vi "NMD Analysis 3.1.vi"(8 "error in (no error)":errorcluster, 11 "Data Cluster In":T1={"Selected File"=path "", "Full Text File"=[], "Data Array"=[], "Times Array"=[], "Sensor Array"=[], "Subset Array"=[], "Smoothness Values"=[], "Sensor Select 1"=refnum, "Sensor Select 2"=refnum, "Sensor Select 3"=refnum, "Sensor Select 4"=refnum, "Start Times"=[], "End Times"=[], "Cursor List"=[{"Name"="Event Marker          ", "Color"=16777200, "Style"=0, "Point Style"=0, "Name Visible"=FALSE, "Allow Drag"=FALSE, "Cursor Mode"=0, "Plot"=0, "Index"=0, "Position"={"X"=4.0, "Y"=1.0}, "X Scale"=0, "Y Scale"=0, "Watch Plots"=[], "Watch All Plots"=FALSE, "Plot Area"=0, "Label Offset"={"X"=-50.0, "Y"=150.0}}, {"Name"="Upper Sensor", "Color"=13816500, "Style"=6, "Point Style"=0, "Name Visible"=FALSE, "Allow Drag"=FALSE, "Cursor Mode"=0, "Plot"=0, "Index"=0, "Position"={"X"=-1.0, "Y"=5.0}, "X Scale"=0, "Y Scale"=0, "Watch Plots"=[], "Watch All Plots"=FALSE, "Plot Area"=0, "Label Offset"={"X"=0.0, "Y"=0.0}}, {"Name"="Lower Sensor", "Color"=13816500, "Style"=6, "Point Style"=0, "Name Visible"=FALSE, "Allow Drag"=FALSE, "Cursor Mode"=0, "Plot"=0, "Index"=0, "Position"={"X"=-1.0, "Y"=30.0}, "X Scale"=0, "Y Scale"=0, "Watch Plots"=[], "Watch All Plots"=FALSE, "Plot Area"=0, "Label Offset"={"X"=0.0, "Y"=0.0}}], "Listbox 1"=refnum, "Listbox 2"=refnum, "Listbox 3"=refnum, "Listbox 4"=refnum, "Labels"=["Why", "is", "this", "still", "not", "built", "into", "Labview?", "This", "is", "shameful."], "Event Array"=[], "Event Names"=[], "Event Times"=[], "Save Plot Button"=refnum, "Sensor Plot Refs"=[], "Selected Event (Title)"="", "Upper Cursor"=0.0, "Lower Cursor"=0.0, "Z Max"=0.0, "Z Min"=0.0}) -> (0 "error out":errorcluster, 3 "Data Cluster Out":T1={"Selected File"=path "", "Full Text File"=[], "Data Array"=[], "Times Array"=[], "Sensor Array"=[], "Subset Array"=[], "Smoothness Values"=[], "Sensor Select 1"=refnum, "Sensor Select 2"=refnum, "Sensor Select 3"=refnum, "Sensor Select 4"=refnum, "Start Times"=[], "End Times"=[], "Cursor List"=[{"Name"="Event Marker          ", "Color"=16777200, "Style"=0, "Point Style"=0, "Name Visible"=FALSE, "Allow Drag"=FALSE, "Cursor Mode"=0, "Plot"=0, "Index"=0, "Position"={"X"=4.0, "Y"=1.0}, "X Scale"=0, "Y Scale"=0, "Watch Plots"=[], "Watch All Plots"=FALSE, "Plot Area"=0, "Label Offset"={"X"=-50.0, "Y"=150.0}}, {"Name"="Upper Sensor", "Color"=13816500, "Style"=6, "Point Style"=0, "Name Visible"=FALSE, "Allow Drag"=FALSE, "Cursor Mode"=0, "Plot"=0, "Index"=0, "Position"={"X"=-1.0, "Y"=5.0}, "X Scale"=0, "Y Scale"=0, "Watch Plots"=[], "Watch All Plots"=FALSE, "Plot Area"=0, "Label Offset"={"X"=0.0, "Y"=0.0}}, {"Name"="Lower Sensor", "Color"=13816500, "Style"=6, "Point Style"=0, "Name Visible"=FALSE, "Allow Drag"=FALSE, "Cursor Mode"=0, "Plot"=0, "Index"=0, "Position"={"X"=-1.0, "Y"=30.0}, "X Scale"=0, "Y Scale"=0, "Watch Plots"=[], "Watch All Plots"=FALSE, "Plot Area"=0, "Label Offset"={"X"=0.0, "Y"=0.0}}], "Listbox 1"=refnum, "Listbox 2"=refnum, "Listbox 3"=refnum, "Listbox 4"=refnum, "Labels"=["Why", "is", "this", "still", "not", "built", "into", "Labview?", "This", "is", "shameful."], "Event Array"=[], "Event Names"=[], "Event Times"=[], "Save Plot Button"=refnum, "Sensor Plot Refs"=[], "Selected Event (Title)"="", "Upper Cursor"=0.0, "Lower Cursor"=0.0, "Z Max"=0.0, "Z Min"=0.0})   [LabVIEW 2020]
uses:
  Controls/DataCluster.ctl
  <vilib>/Utility/miscctls.llb/LVCursorListTypeDef.ctl
  Controls/SPARC Analysis States.ctl
  <userlib>/_OpenG.lib/file/file.llb/File Exists - Scalar__ogtk.vi
panel:
  out "NMD Plot":picture
  out "Saving":bool
  out "Analyzing":bool
  out "Segmenting":bool
  out "Selected Segment":dbl[][](graph)
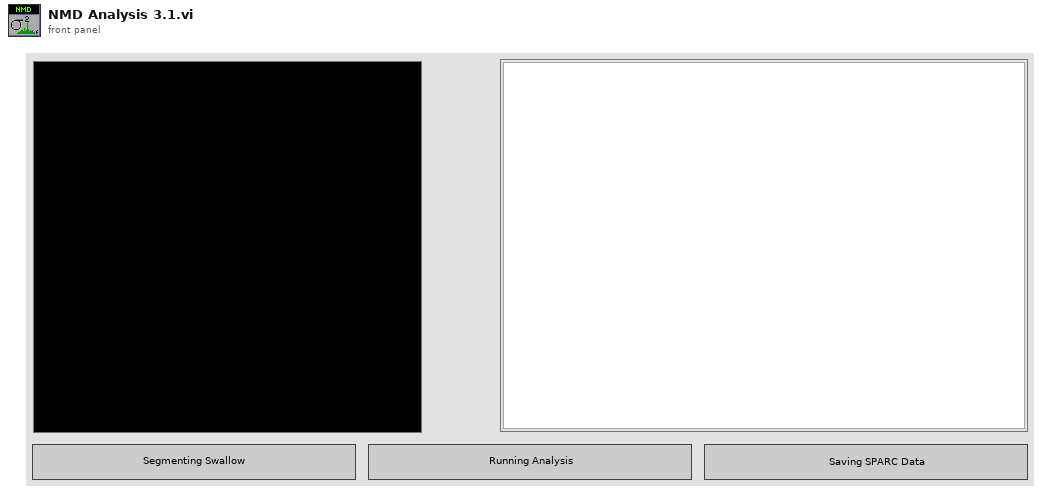
[diagram p1: front panel]
types:
  T1 = typedef "DataCluster.ctl" = cluster{"Selected File":path, "Full Text File":string[][], "Data Array":dbl[][], "Times Array":dbl[], "Sensor Array":dbl[], "Subset Array":dbl[][], "Smoothness Values":dbl[], "Sensor Select 1":refnum<vi>, "Sensor Select 2":refnum<vi>, "Sensor Select 3":refnum<vi>, "Sensor Select 4":refnum<vi>, "Start Times":dbl[], "End Times":dbl[], "Cursor List":T2, "Listbox 1":refnum<vi>, "Listbox 2":refnum<vi>, "Listbox 3":refnum<vi>, "Listbox 4":refnum<vi>, "Labels":string[], "Event Array":dbl[][], "Event Names":string[], "Event Times":dbl[], "Save Plot Button":refnum<vi>, "Sensor Plot Refs":refnum<vi>[], "Selected Event (Title)":string, "Upper Cursor":dbl, "Lower Cursor":dbl, "Z Max":dbl, "Z Min":dbl}
  T2 = typedef "LVCursorListTypeDef.ctl" = cluster{"Name":string, "Color":u32, "Style":u8, "Point Style":u8, "Name Visible":bool, "Allow Drag":bool, "Cursor Mode":u32, "Plot":i32, "Index":i32, "Position":cluster{"X":dbl, "Y":dbl}, "X Scale":u32, "Y Scale":u32, "Watch Plots":i32[], "Watch All Plots":bool, "Plot Area":i32, "Label Offset":cluster{"X":dbl, "Y":dbl}}[]
  T3 = typedef "SPARC Analysis States.ctl" = enum16{"Segment", "Analyze", "Save"}
  T4 = cluster{"Cursor List[0]":cluster{"Name":string, "Color":u32, "Style":u8, "Point Style":u8, "Name Visible":bool, "Allow Drag":bool, "Cursor Mode":u32, "Plot":i32, "Index":i32, "Position":cluster{"X":dbl, "Y":dbl}, "X Scale":u32, "Y Scale":u32, "Watch Plots":i32[], "Watch All Plots":bool, "Plot Area":i32, "Label Offset":cluster{"X":dbl, "Y":dbl}}, "Cursor List[1]":cluster{"Name":string, "Color":u32, "Style":u8, "Point Style":u8, "Name Visible":bool, "Allow Drag":bool, "Cursor Mode":u32, "Plot":i32, "Index":i32, "Position":cluster{"X":dbl, "Y":dbl}, "X Scale":u32, "Y Scale":u32, "Watch Plots":i32[], "Watch All Plots":bool, "Plot Area":i32, "Label Offset":cluster{"X":dbl, "Y":dbl}}, "Cursor List[2]":cluster{"Name":string, "Color":u32, "Style":u8, "Point Style":u8, "Name Visible":bool, "Allow Drag":bool, "Cursor Mode":u32, "Plot":i32, "Index":i32, "Position":cluster{"X":dbl, "Y":dbl}, "X Scale":u32, "Y Scale":u32, "Watch Plots":i32[], "Watch All Plots":bool, "Plot Area":i32, "Label Offset":cluster{"X":dbl, "Y":dbl}}, "Cursor List[3]":cluster{"Name":string, "Color":u32, "Style":u8, "Point Style":u8, "Name Visible":bool, "Allow Drag":bool, "Cursor Mode":u32, "Plot":i32, "Index":i32, "Position":cluster{"X":dbl, "Y":dbl}, "X Scale":u32, "Y Scale":u32, "Watch Plots":i32[], "Watch All Plots":bool, "Plot Area":i32, "Label Offset":cluster{"X":dbl, "Y":dbl}}, "Cursor List[4]":cluster{"Name":string, "Color":u32, "Style":u8, "Point Style":u8, "Name Visible":bool, "Allow Drag":bool, "Cursor Mode":u32, "Plot":i32, "Index":i32, "Position":cluster{"X":dbl, "Y":dbl}, "X Scale":u32, "Y Scale":u32, "Watch Plots":i32[], "Watch All Plots":bool, "Plot Area":i32, "Label Offset":cluster{"X":dbl, "Y":dbl}}, "Cursor List[5]":cluster{"Name":string, "Color":u32, "Style":u8, "Point Style":u8, "Name Visible":bool, "Allow Drag":bool, "Cursor Mode":u32, "Plot":i32, "Index":i32, "Position":cluster{"X":dbl, "Y":dbl}, "X Scale":u32, "Y Scale":u32, "Watch Plots":i32[], "Watch All Plots":bool, "Plot Area":i32, "Label Offset":cluster{"X":dbl, "Y":dbl}}, "Cursor List[6]":cluster{"Name":string, "Color":u32, "Style":u8, "Point Style":u8, "Name Visible":bool, "Allow Drag":bool, "Cursor Mode":u32, "Plot":i32, "Index":i32, "Position":cluster{"X":dbl, "Y":dbl}, "X Scale":u32, "Y Scale":u32, "Watch Plots":i32[], "Watch All Plots":bool, "Plot Area":i32, "Label Offset":cluster{"X":dbl, "Y":dbl}}, "Cursor List[7]":cluster{"Name":string, "Color":u32, "Style":u8, "Point Style":u8, "Name Visible":bool, "Allow Drag":bool, "Cursor Mode":u32, "Plot":i32, "Index":i32, "Position":cluster{"X":dbl, "Y":dbl}, "X Scale":u32, "Y Scale":u32, "Watch Plots":i32[], "Watch All Plots":bool, "Plot Area":i32, "Label Offset":cluster{"X":dbl, "Y":dbl}}, "Cursor List[8]":cluster{"Name":string, "Color":u32, "Style":u8, "Point Style":u8, "Name Visible":bool, "Allow Drag":bool, "Cursor Mode":u32, "Plot":i32, "Index":i32, "Position":cluster{"X":dbl, "Y":dbl}, "X Scale":u32, "Y Scale":u32, "Watch Plots":i32[], "Watch All Plots":bool, "Plot Area":i32, "Label Offset":cluster{"X":dbl, "Y":dbl}}}
  T5 = cluster{"Name":string, "Color":u32, "Style":u8, "Point Style":u8, "Name Visible":bool, "Allow Drag":bool, "Cursor Mode":u32, "Plot":i32, "Index":i32, "Position":cluster{"X":dbl, "Y":dbl}, "X Scale":u32, "Y Scale":u32, "Watch Plots":i32[], "Watch All Plots":bool, "Plot Area":i32, "Label Offset":cluster{"X":dbl, "Y":dbl}}[]
  T6 = enum16{"open", "replace", "create", "open or create", "replace or create", "replace or create with confirmation"}
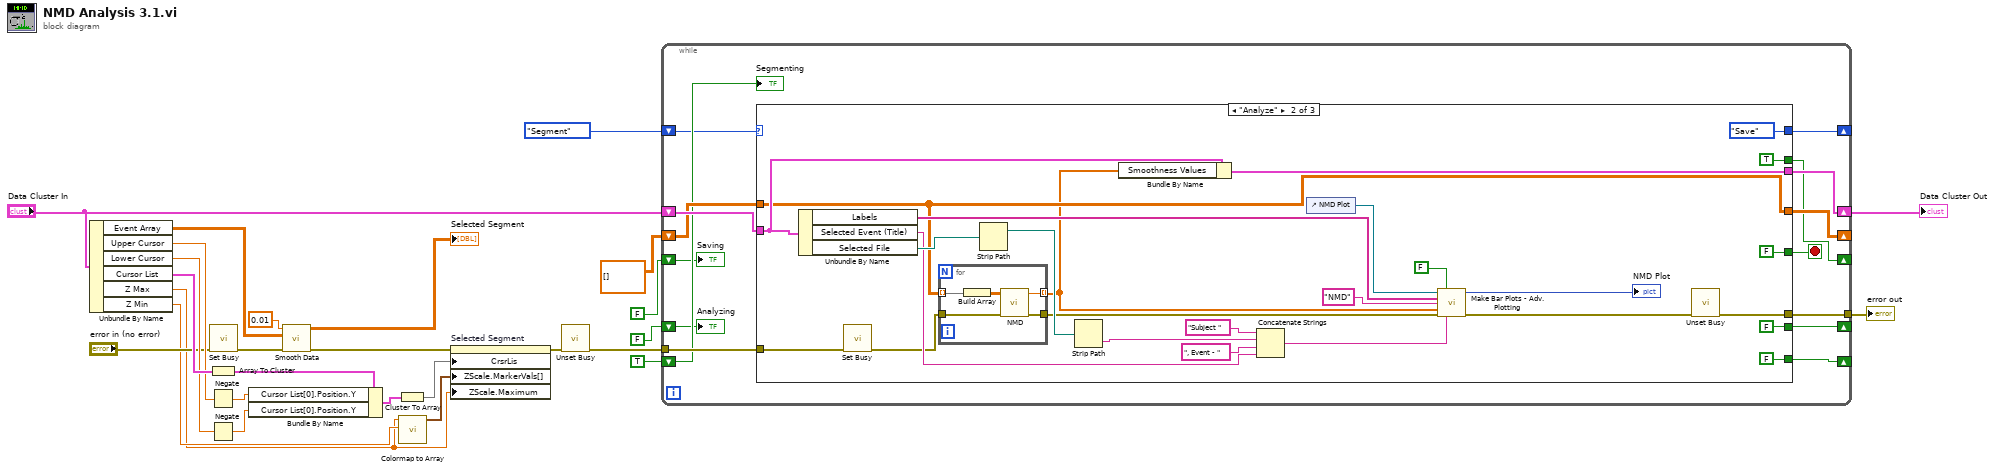
[diagram p0: block diagram]
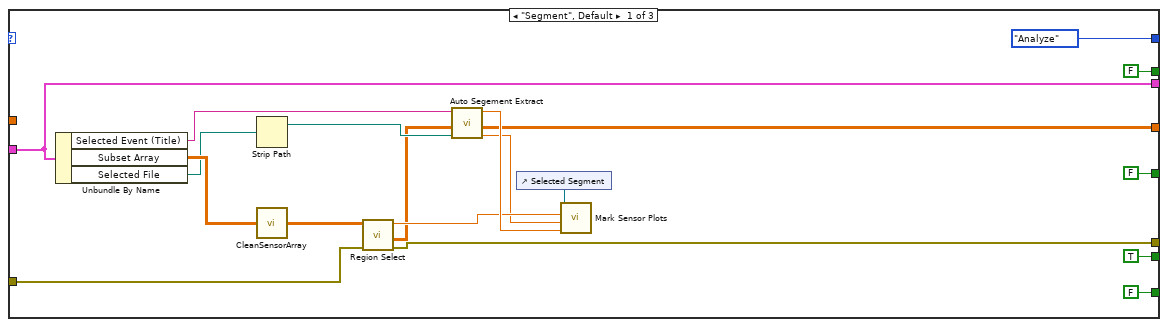
[diagram p2: hidden frame]
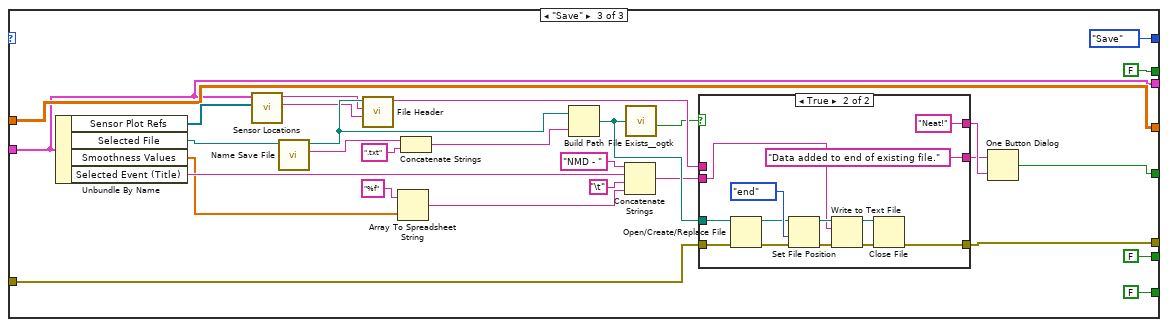
[diagram p3: hidden frame]
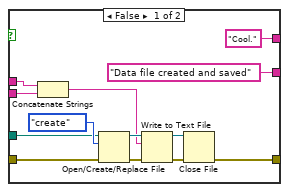
[diagram p4: hidden frame]
diagram:
  n1 = Unbundle By Name("Data Cluster In") -> ("Event Array"=w27:dbl[][], "Upper Cursor"=w18:dbl, "Lower Cursor"=w17:dbl, "Cursor List"=w23:T2, "Z Max"=w1:dbl, "Z Min"=w2:dbl)
  n2 = Array To Cluster(array=w23) -> (cluster=w22:T4)
  n3 = Negate(x=w18) -> (-x=w20:dbl)
  n4 = Negate(x=w17) -> (-x=w19:dbl)
  n5 = call <vilib>:"Set Busy.vi"("error in (no error)"="error in (no error)") -> ("error out"=w14:errorcluster)  [unwired: 9 in, 1 out]
  n6 = Bundle By Name(cluster=w22, "Cursor List[0].Position.Y"=w20, "Cursor List[0].Position.Y"=w19) -> (w21:T4)
  n7 = call "Smooth Data.vi"("error in (no error)"=w14, "Data Array"=w27, "dt"=0.01) -> ("error out"=w7:errorcluster, "Resampled Array"=→"Selected Segment":dbl[][])  [unwired: 7 in]
  n8 = Cluster To Array(cluster=w21) -> (array=w8:T5)
  n9 = call "Colormap to Array.vi"("Min Pressure"=w2, "Max Pressure"=w1) -> ("Z Scale.Marker Values[]"=w5:cluster{dbl, u32}[])  [unwired: 9 in]
  n10 = property on="Selected Segment" class="IntGraph (strict)"(error in=w7, "CrsrLis"=w8, "ZScale.MarkerVals[]"=w5, "ZScale.Maximum"=w1) -> (error out=w6:errorcluster)  [unwired: 1 in, 1 out]
  n11 = call <vilib>:"Unset Busy.vi"("error in (no error)"=w6) -> ("error out"=w13:errorcluster)  [unwired: 10 in]
  n12 = while {
    tunnel: w13 -> [w40]
    tunnel: [w41] -> w24
    shift-right: [w42] -> _
    shift-left: dbl[][] [] ("Trimmed Segment") -> [w38]
    shift-right: [w36] -> w3
    shift-left: "Data Cluster In" -> [w39]
    shift-right: [w32] -> _
    shift-left: TRUE -> [w35]
    shift-right: [w31] -> _
    shift-left: FALSE -> [w34]
    shift-right: [w30] -> _
    shift-left: FALSE -> [w33]
    shift-right: [w28] -> _
    shift-left: SPARC_Analysis_States."Segment" -> [w29]
    stop <- w37 stop-if-true
    n13 = case shown="\"Analyze\"" w29 {
      tunnel: w40 -> [w52 w71 w102]
      tunnel: w39 -> [w48 w74 w98]
      tunnel: [w51 w64 w99] -> w42
      tunnel: [w50 w73 w100] -> w41
      tunnel: w38 -> [_ w64 w99]
      tunnel: [w48 w75 w98] -> w36
      tunnel: [FALSE ("true") FALSE ("true") w101] -> w37
      tunnel: [FALSE FALSE FALSE] -> w32
      tunnel: [TRUE FALSE FALSE] -> w31
      tunnel: [FALSE TRUE FALSE] -> w30
      tunnel: [SPARC_Analysis_States."Analyze" SPARC_Analysis_States."Save" SPARC_Analysis_States."Save"] -> w28
      frame "Segment", Default {
        n14 = Unbundle By Name(w48) -> ("Selected Event (Title)"=w56:string, "Subset Array"=w54:dbl[][], "Selected File"=w53:path)
        n15 = Strip Path(path=w53) -> (stripped path=w58:path)  [unwired: 1 out]
        n16 = call "CleanSensorArray.vi"("Sensor Data Array"=w54) -> ("Clean Array"=w55:dbl[][])  [unwired: 4 in]
        n17 = call "Region Select.vi"("Error In"=w52, "Sensor Data Array"=w55) -> ("Error Out"=w50:errorcluster, "Trimmed Event"=w57:dbl[][], "Segement Start"=w60:dbl)  [unwired: 7 in]
        n18 = call "Auto Segement Extract.vi"("Save Path"=w58, "Sensor Data Array"=w57, "Title"=w56) -> ("End"=w43:dbl, "Trimmed Segment"=w51:dbl[][], "Start"=w61:dbl)  [unwired: 1 in, 1 out]
        n19 = control-ref of="Selected Segment"() -> (w59:refnum<vi>)
        n20 = call "Mark Sensor Plots.vi"("Segment Select Ref"=w59, "Segement Start"=w60, "End"=w43, "Start"=w61) -> ()  [unwired: 7 in]
      }
      frame "Analyze" {
        n21 = Unbundle By Name(w74) -> ("Labels"=w81:string[], "Selected Event (Title)"=w83:string, "Selected File"=w84:path)
        n22 = call <vilib>:"Set Busy.vi"("error in (no error)"=w71) -> ("error out"=w65:errorcluster)  [unwired: 9 in, 1 out]
        n23 = for {
          tunnel: w64 -> [w90] mode=indexing
          tunnel: [w92] -> w80
          tunnel: w65 -> [w91]
          tunnel: [w88] -> w63 mode=indexing
          n24 = Build Array(w90) -> (w89:dbl[][])
          n25 = call "NMD.vi"("error in"=w91, "RoI"=w89) -> ("error out"=w92:errorcluster, "NMD"=w88:dbl)  [unwired: 8 in]
        }
        n26 = Strip Path(path=w84) -> (stripped path=w85:path)  [unwired: 1 out]
        n27 = Strip Path(path=w85) -> (name=w86:string)  [unwired: 1 out]
        n28 = Bundle By Name(cluster=w74, "Smoothness Values"=w63) -> (w75:T1)
        n29 = Concatenate Strings("Subject " ("string"), w86, ", Event - " ("string"), w83) -> (w82:string)
        n30 = control-ref of="NMD Plot"() -> (w79:refnum<vi>)
        n31 = call "Make Bar Plots - Adv. Plotting.vi"("Picture in"=w79, "Save Plot?"=FALSE, "Labels"=w81, "Legend Title"="NMD", "SPARC"=w63, "error in (no error)"=w80, "Title"=w82) -> ("Picture"=→"NMD Plot":picture, "error out"=w87:errorcluster)  [unwired: 7 in]
        n32 = call <vilib>:"Unset Busy.vi"("error in (no error)"=w87) -> ("error out"=w73:errorcluster)  [unwired: 10 in]
      }
      frame "Save" {
        n33 = Unbundle By Name(w98) -> ("Sensor Plot Refs"=w109:refnum<vi>[], "Selected File"=w108:path, "Smoothness Values"=w93:dbl[], "Selected Event (Title)"=w111:string)
        n34 = call "Sensor Locations.vi"("Ref Array"=w109, "Data Cluster In"=w98) -> ("Sensors"=w114:string, "Locations"=w113:string)  [unwired: 8 in]
        n35 = call "Name Save File.vi"("Selected File"=w108) -> ("Name"=w116:string, "stripped path"=w117:path)  [unwired: 9 in]
        n36 = call "File Header.vi"("Sensors"=w114, "Locations"=w113, "Stripped Path"=w117) -> ("File Header"=w115:string)  [unwired: 8 in]
        n37 = Array To Spreadsheet String(array=w93, 3:"%f" ("format string")) -> (spreadsheet string=w112:string)  [unwired: 1 in]
        n38 = Concatenate Strings(w116, ".txt" ("string")) -> (w107:string)
        n39 = Build Path(base path=w117, name or relative path=w107) -> (appended path=w121:path)
        n40 = Concatenate Strings("NMD - " ("string"), w111, "\t", w112) -> (w120:string)
        n41 = call-poly <userlib>:"File Exists__ogtk.vi"("file path"=w121) -> ("exists"=w110:bool)  [unwired: 6 in, 1 out]
        n42 = case shown="True" w110 {
          tunnel: w115 -> [w125 _]
          tunnel: w121 -> [w133 w147]
          tunnel: [w129 w141] -> w100
          tunnel: ["Data file created and saved" "Data added to end of existing file."] -> w118
          tunnel: ["Cool." "Neat!"] -> w119
          tunnel: w120 -> [w122 w136]
          tunnel: w102 -> [w123 w135]
          frame False {
            n43 = Concatenate Strings(w125, w122) -> (w124:string)
            n44 = Open/Create/Replace File(file path (use dialog)=w133, error in=w123, operation (0:open)=T6."create") -> (refnum out=w132:refnum<file>, error out=w131:errorcluster)  [unwired: 3 in, 1 out]
            n45 = Write to Text File(file (use dialog)=w132, text=w124, error in=w131) -> (refnum out=w128:refnum<file>, error out=w130:errorcluster)  [unwired: 1 in, 1 out]
            n46 = Close File(refnum=w128, error in=w130) -> (error out=w129:errorcluster)  [unwired: 1 out]
          }
          frame True {
            n47 = Open/Create/Replace File(file path (use dialog)=w147, error in=w135) -> (refnum out=w145:refnum<file>, error out=w144:errorcluster)  [unwired: 4 in, 1 out]
            n48 = Set File Position(refnum=w145, from (0:start)=enum16{"start", "end", "current"}."end", error in=w144) -> (refnum out=w140:refnum<file>, error out=w143:errorcluster)  [unwired: 1 in]
            n49 = Write to Text File(file (use dialog)=w140, text=w136, error in=w143) -> (refnum out=w139:refnum<file>, error out=w142:errorcluster)  [unwired: 1 in, 1 out]
            n50 = Close File(refnum=w139, error in=w142) -> (error out=w141:errorcluster)  [unwired: 1 out]
          }
        }
        n51 = One Button Dialog(message=w118, button name ("OK")=w119) -> (true=w101:bool)
      }
    }
    "Saving" <- w33
    "Analyzing" <- w34
    "Segmenting" <- w35
  }
  "error out" <- w24
  "Data Cluster Out" <- w3
